vi "Write Command ID.vi"(8 "error in (no error)":errorcluster, 10 "Command ID":u16, 11 "Packet in":refnum<class "Packet.lvclass">) -> (0 "error out":errorcluster, 3 "Packet out":refnum<class "Packet.lvclass">)   [LabVIEW 2020, in "Communication Classes.lvlib" / "Packet.lvclass"]
uses:
  Packet.lvclass
  Packet.lvclass/Packet.ctl
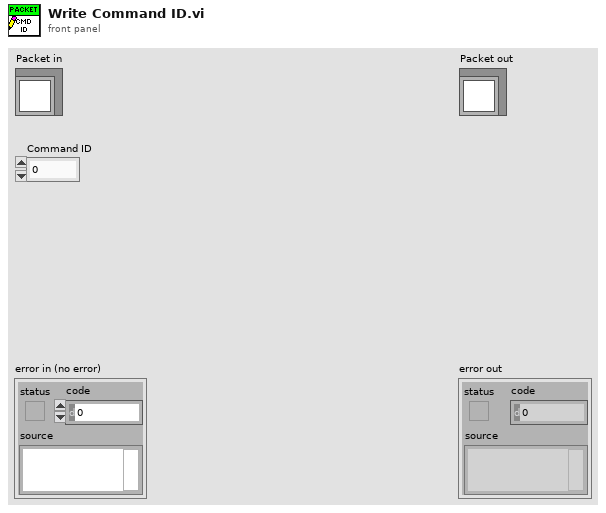
[diagram p1: front panel]
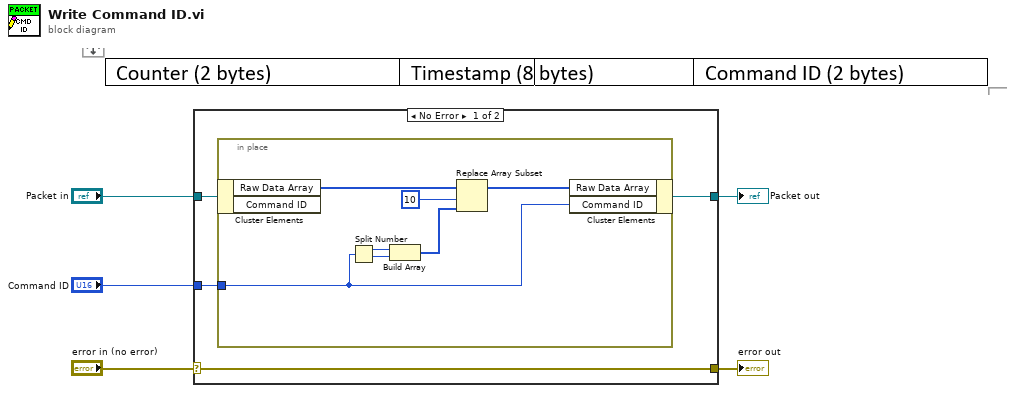
[diagram p0: block diagram]
diagram:
  n1 = case shown="No Error" "error in (no error)" {
    selector: "error in (no error)" -> [w9 w17]
    tunnel: [w9 w17] -> w4
    tunnel: [w6 w18] -> w2
    tunnel: "Packet in" -> [w8 w18]
    tunnel: "Command ID" -> [w7 _]
    frame No Error {
      n2 = in-place {
        in-place-border: w7 -> [w14]
        n3 = in-place-cluster #1(w8) -> ("Raw Data Array"=w16:u8[])  [unwired: 1 out]
        n4 = Split Number(x=w14) -> (hi(x)=w13:u8, lo(x)=w12:u8)
        n5 = Build Array(w13, w12) -> (w11:u8[])
        n6 = Replace Array Subset "Replace Array Subset"(array=w16, new element=w11, index=10) -> (w15:u8[])
        n7 = in-place-cluster #1("Raw Data Array"=w15, "Command ID"=w14) -> (w6:refnum<class "Packet.lvclass">)
      }
    }
    frame Error {
    }
  }
  "error out" <- w4
  "Packet out" <- w2
